vi "test_DiscoverDevices.vi"(8 "error in":errorcluster) -> (0 "error out":errorcluster)   [LabVIEW 2023, in "horiba.test.lvlib"]
doc: "_____\nCreated using DQMH Event Scripter 7.0.1.1316."
uses:
  horiba.test.lvlib
  Classes/Mono/Monochromator.lvclass
  Classes/CCD/CCD.lvclass
  <vilib>/addons/_JKI Toolkits/Caraya/classes/Assert/Assert Equal Value and Type_Variant.vi
  Classes/DeviceManager/DeviceManager.lvlib
  <vilib>/addons/_JKI Toolkits/Caraya/classes/Test/Test.lvclass
  <vilib>/addons/_JKI Toolkits/Caraya/classes/Assert/Assert.lvclass
  C:/Projects/Horiba/horiba-labview-sdk/Source/Classes/GenericDevice/GenericDevice.lvclass
  C:/Projects/Horiba/horiba-labview-sdk/Source/Classes/Mono/Monochromator.lvclass
  C:/Projects/Horiba/horiba-labview-sdk/Source/Classes/CCD/CCD.lvclass
  Classes/SCD/SCD.lvclass
  C:/Projects/Horiba/horiba-labview-sdk/Source/Classes/SCD/SCD.lvclass
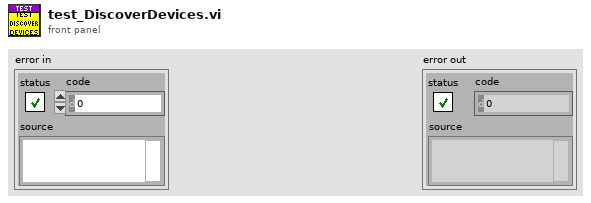
[diagram p1: front panel]
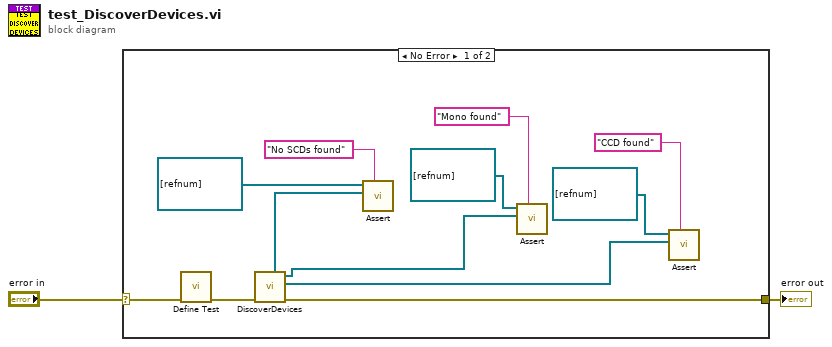
[diagram p0: block diagram]
diagram:
  n1 = case shown="No Error" "error in" {
    selector: "error in" -> [w14 w15]
    tunnel: [w13 w15] -> w1
    frame No Error {
      n2 = call <vilib>:"Define Test.vi"("error in (no error)"=w14) -> ("error out"=w12:errorcluster)  [unwired: 9 in, 1 out]
      n3 = call "DiscoverDevices.vi"("error in"=w12) -> ("error out"=w13:errorcluster, "CCDs"=w4:refnum<class "CCD.lvclass">[], "Monos"=w8:refnum<class "Monochromator.lvclass">[], "SCDs"=w10:refnum<class "SCD.lvclass">[])  [unwired: 6 in, 1 out]
      n4 = call-poly <vilib>:"Assert.vi"("Label"="No SCDs found", "Y"=w10, "X"=refnum<class "SCD.lvclass">[] [refnum] ("SCDs")) -> ()  [unwired: 7 in, 2 out]
      n5 = call-poly <vilib>:"Assert.vi"("Label"="Mono found", "Y"=w8, "X"=refnum<class "Monochromator.lvclass">[] [refnum] ("Monos")) -> ()  [unwired: 7 in, 2 out]
      n6 = call-poly <vilib>:"Assert.vi"("Label"="CCD found", "Y"=w4, "X"=refnum<class "CCD.lvclass">[] [refnum] ("CCDs")) -> ()  [unwired: 7 in, 2 out]
    }
    frame Error {
    }
  }
  "error out" <- w1
